vi "XWPF Reader - Tests.vi"(8 "error in (no error)":errorcluster) -> (0 "error out":errorcluster)   [LabVIEW 2017]
uses:
  <vilib>/addons/_JKI Toolkits/Caraya/classes/Assert/Assert Not Error.vi
  <vilib>/addons/_JKI Toolkits/Caraya/classes/Assert/Assert True.vi
  src/LabVIEW NPOI/xwpfReader/xwpfReader.lvclass
  <vilib>/addons/_JKI Toolkits/Caraya/classes/Test/Test.lvclass
  <vilib>/addons/_JKI Toolkits/Caraya/classes/Assert/Assert.lvclass
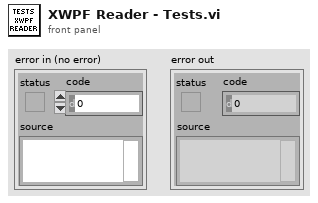
[diagram p1: front panel]
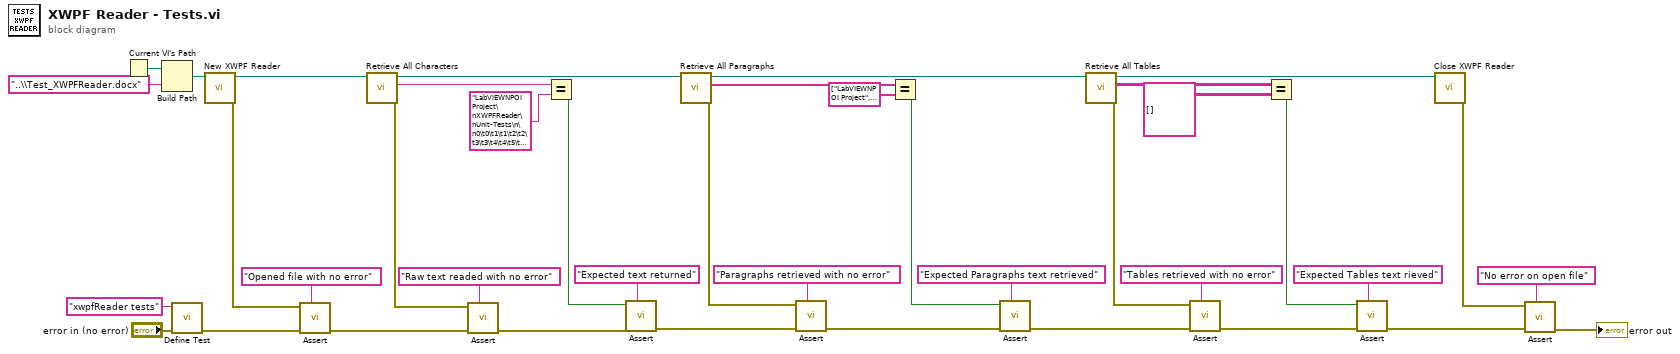
[diagram p0: block diagram]
diagram:
  n1 = Current VI's Path() -> (path=w36:path)
  n2 = Build Path(base path=w36, name or relative path="..\\Test_XWPFReader.docx" ("string")) -> (appended path=w34:path)
  n3 = call <vilib>:"Define Test.vi"("error in (no error)"="error in (no error)", "Label (VI Title)"="xwpfReader tests") -> ("error out"=w31:errorcluster)  [unwired: 9 in]
  n4 = call "New XWPF Reader.vi"("XWPF File Path"=w34) -> ("error out"=w30:errorcluster, "xwpfReader out"=w39:refnum<class "xwpfReader.lvclass">)  [unwired: 9 in]
  n5 = call-poly <vilib>:"Assert.vi"("Label"="Opened file with no error", "error in (no error)"=w31, "Not Error?"=w30) -> ("error out"=w23:errorcluster)  [unwired: 8 in]
  n6 = call "Retrieve All Characters.vi"("xwpfReader in"=w39) -> ("error out"=w24:errorcluster, "All Characters"=w22:string, "xwpfReader out"=w40:refnum<class "xwpfReader.lvclass">)  [unwired: 8 in]
  n7 = call-poly <vilib>:"Assert.vi"("Label"="Raw text readed with no error", "error in (no error)"=w23, "Not Error?"=w24) -> ("error out"=w19:errorcluster)  [unwired: 8 in]
  n8 = Equal?(x=w22, y="LabVIEWNPOI Project\nXWPFReader\nUnit-Tests\n\n0\t0\t1\t1\t2\t2\t3\t3\t4\t4\t5\t5\t6\t6\t7\t7\t8\t8\t9\t9\n0\t0\t1\t1\t2\t2\t3\t3\t4\t4\t5\t5\t6\t6\t7\t7\t8\t8\t9\t9\n\n" ("All Characters")) -> (x = y?=w18:bool)
  n9 = call-poly <vilib>:"Assert.vi"("Label"="Expected text returned", "error in (no error)"=w19, "True?"=w18) -> ("error out"=w17:errorcluster)  [unwired: 8 in]
  n10 = call "Retrieve All Paragraphs.vi"("xwpfReader in"=w40) -> ("error out"=w16:errorcluster, "Paragraphs"=w21:string[], "xwpfReader out"=w38:refnum<class "xwpfReader.lvclass">)  [unwired: 8 in]
  n11 = call-poly <vilib>:"Assert.vi"("Label"="Paragraphs retrieved with no error", "error in (no error)"=w17, "Not Error?"=w16) -> ("error out"=w14:errorcluster)  [unwired: 8 in]
  n12 = Equal?(x=w21, y=string[] ["LabVIEWNPOI Project", "XWPFReader", "Unit-Tests", ""] ("Paragraphs")) -> (x = y?=w13:bool)
  n13 = call-poly <vilib>:"Assert.vi"("Label"="Expected Paragraphs text retrieved", "error in (no error)"=w14, "True?"=w13) -> ("error out"=w12:errorcluster)  [unwired: 8 in]
  n14 = call "Retrieve All Tables.vi"("xwpfReader in"=w38) -> ("error out"=w11:errorcluster, "Tables"=w6:string[][][], "xwpfReader out"=w37:refnum<class "xwpfReader.lvclass">)  [unwired: 8 in]
  n15 = call-poly <vilib>:"Assert.vi"("Label"="Tables retrieved with no error", "error in (no error)"=w12, "Not Error?"=w11) -> ("error out"=w9:errorcluster)  [unwired: 8 in]
  n16 = Equal?(x=w6, y=string[][][] [] ("Tables")) -> (x = y?=w5:bool)
  n17 = call-poly <vilib>:"Assert.vi"("Label"="Expected Tables text rieved", "error in (no error)"=w9, "True?"=w5) -> ("error out"=w8:errorcluster)  [unwired: 8 in]
  n18 = call "Close XWPF Reader.vi"("xwpfReader in"=w37) -> ("error out"=w7:errorcluster)  [unwired: 9 in, 1 out]
  n19 = call-poly <vilib>:"Assert.vi"("Label"="No error on open file", "error in (no error)"=w8, "Not Error?"=w7) -> ("error out"=→"error out":errorcluster)  [unwired: 8 in]
